vi "Set KH BW Filter.vi"(8 "error in (no error)":errorcluster, 10 "Bandwidth Filter":T5=enum."ON", 11 "KH Cluster":T1) -> (0 "error out":errorcluster, 3 "KH Cluster out":T1)   [LabVIEW 2016, in "Control Experiment UI.lvclass"]
uses:
  Control Experiment UI.lvclass
  <userlib>/LevyLab/Krohn Hite 7008/typedefs/Filter-Enum.ctl
  Typedefs/KH Cluster--Cluster.ctl
  <userlib>/LevyLab/Krohn Hite 7008/typedefs/SetAll-Cluster.ctl
  <userlib>/LevyLab/Krohn Hite 7008/typedefs/Channel-Enum.ctl
  <userlib>/LevyLab/Krohn Hite 7008/typedefs/Gain-Enum.ctl
  <userlib>/LevyLab/Krohn Hite 7008/typedefs/Shunt-Enum.ctl
  <userlib>/LevyLab/Krohn Hite 7008/typedefs/Coupling-Enum.ctl
  <userlib>/LevyLab/Krohn Hite 7008/typedefs/Input Configuration-Enum.ctl
  <userlib>/LevyLab/Krohn Hite 7008/Instrument.KH7008.lvclass
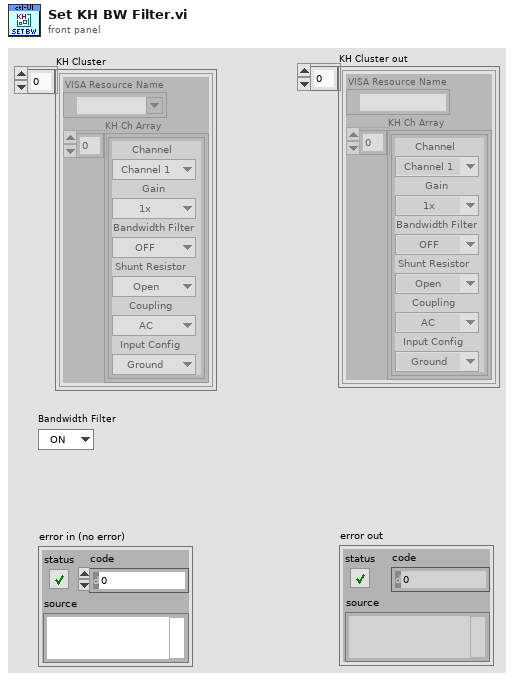
[diagram p1: front panel]
types:
  T1 = typedef "KH Cluster--Cluster.ctl" = cluster{"VISA Resource Name":refnum<visa-resource-name>, "KH Ch Array":T2[]}[]
  T2 = typedef "Instrument.KH7008.lvclass/SetAll-Cluster.ctl" = cluster{"Channel":T3, "Gain":T4, "Bandwidth Filter":T5, "Shunt Resistor":T6, "Coupling":T7, "Input Config":T8}
  T3 = typedef "Instrument.KH7008.lvclass/Channel-Enum.ctl" = enum16{"Channel 1", "Channel 2", "Channel 3", "Channel 4", "Channel 5", "Channel 6", "Channel 7", "Channel 8"}
  T4 = typedef "Instrument.KH7008.lvclass/Gain-Enum.ctl" = enum16{"1x", "10x", "100x", "1000x"}
  T5 = typedef "Instrument.KH7008.lvclass/Filter-Enum.ctl" = enum16{"OFF", "ON"}
  T6 = typedef "Instrument.KH7008.lvclass/Shunt-Enum.ctl" = enum16{"Open", "50 Ohms", "500 Ohms", "5k Ohms", "50k Ohms", "10M Ohm"}
  T7 = typedef "Instrument.KH7008.lvclass/Coupling-Enum.ctl" = enum16{"AC", "DC"}
  T8 = typedef "Instrument.KH7008.lvclass/Input Configuration-Enum.ctl" = enum16{"Ground", "SE+ (-gnd)", "SE- (+gnd)", "Differential"}
  T9 = cluster{"VISA Resource Name":refnum<visa-resource-name>, "KH Ch Array":T2[]}
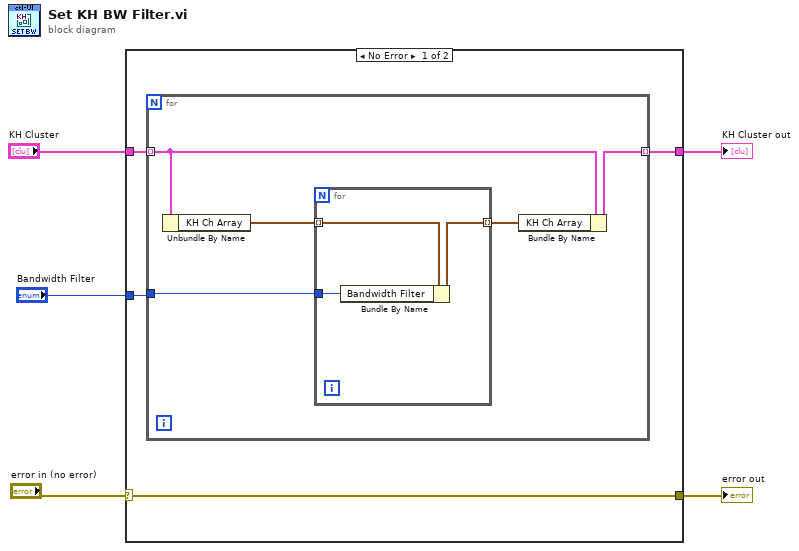
[diagram p0: block diagram]
diagram:
  n1 = case shown="No Error" "error in (no error)" {
    selector: "error in (no error)" -> [w7 w18]
    tunnel: "Bandwidth Filter" -> [w9 _]
    tunnel: "KH Cluster" -> [w8 w19]
    tunnel: [w7 w18] -> w2
    tunnel: [w6 w19] -> w1
    frame No Error {
      n2 = for {
        tunnel: w8 -> [w14] mode=indexing
        tunnel: [w13] -> w6 mode=indexing
        tunnel: w9 -> [w12]
        n3 = Unbundle By Name(w14) -> ("KH Ch Array"=w11:T2[])
        n4 = for {
          tunnel: w12 -> [w17]
          tunnel: w11 -> [w16] mode=indexing
          tunnel: [w15] -> w10 mode=indexing
          n5 = Bundle By Name(cluster=w16, "Bandwidth Filter"=w17) -> (w15:T2)
        }
        n6 = Bundle By Name(cluster=w14, "KH Ch Array"=w10) -> (w13:T9)
      }
    }
    frame Error {
    }
  }
  "KH Cluster out" <- w1
  "error out" <- w2
